vi "Cam prepare task.vi"(7 "save folder":path, 8 "error in (no error)":errorcluster, 10 "Cam task parameters":T1, 11 "Camera in":refnum<class "Camera.lvclass">) -> (0 "error out":errorcluster, 3 "Camera out":refnum<class "Camera.lvclass">)   [LabVIEW 2021, in "Camera.lvlib" / "Camera.lvclass"]
uses:
  Camera.lvclass
  C:/Program Files (x86)/National Instruments/LabVIEW 2021/vi.lib/ActorFramework/Actor/Actor.lvclass
  Cam task parameters.ctl
  Camera.lvclass/Camera.ctl
  <vilib>/ActorFramework/Actor/Actor.lvclass/Actor.ctl
  Main_Control/Main_Control Messages/UI change exposure time Msg/UI change exposure time Msg.lvclass/UI change exposure time Msg.ctl
  <vilib>/ActorFramework/Message Enqueuer/Message Enqueuer.lvclass/Message Enqueuer.ctl
  Main_Control/Main_Control/notifications.ctl
  Main_Control/Main_Control Messages/UI notifier Msg/UI notifier Msg.lvclass/UI notifier Msg.ctl
  <vilib>/ActorFramework/Message Enqueuer/Enqueue.vi
  Main_Control/Main_Control Messages/UI change exposure time Msg/UI change exposure time Msg.lvclass
  C:/Program Files (x86)/National Instruments/LabVIEW 2021/vi.lib/ActorFramework/Message/Message.lvclass
  Main_Control/Main_Control Messages/UI notifier Msg/UI notifier Msg.lvclass
  <vilib>/ActorFramework/Message Priority Queue/Priority Enqueue.vi
  <vilib>/ActorFramework/Actor/Actor.lvclass
  Main_Control/Main_Control/Main_Control.lvclass
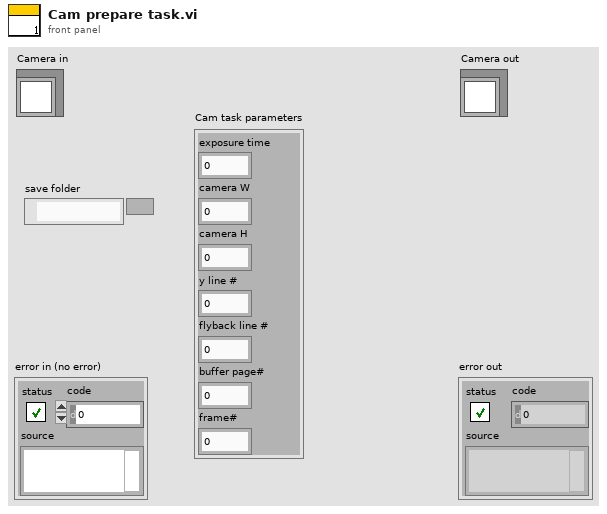
[diagram p1: front panel]
types:
  T1 = typedef "Camera.lvlib/Camera.lvclass/Cam task parameters.ctl" = cluster{"exposure time":dbl, "camera W":dbl, "camera H":dbl, "y line #":dbl, "flyback line #":dbl, "buffer page#":dbl, "frame#":dbl}
  T2 = cluster{"Horizontal Offset":i32, "Vertical Offset":i32, "Horizontal Size":i32, "Vertical Size":i32}
  T3 = typedef "Main_Control.lvlib/Main_Control.lvclass/notifications.ctl" = enum16{"cam 1 frame skkipped", "cam finish", "cam started", "cam stopped", "cam updated", "ni started", "ni stopped", "ni updated"}
  T4 = cluster{"Full Height":dbl, "Full Width":dbl, "Output Trigger Port":dbl}
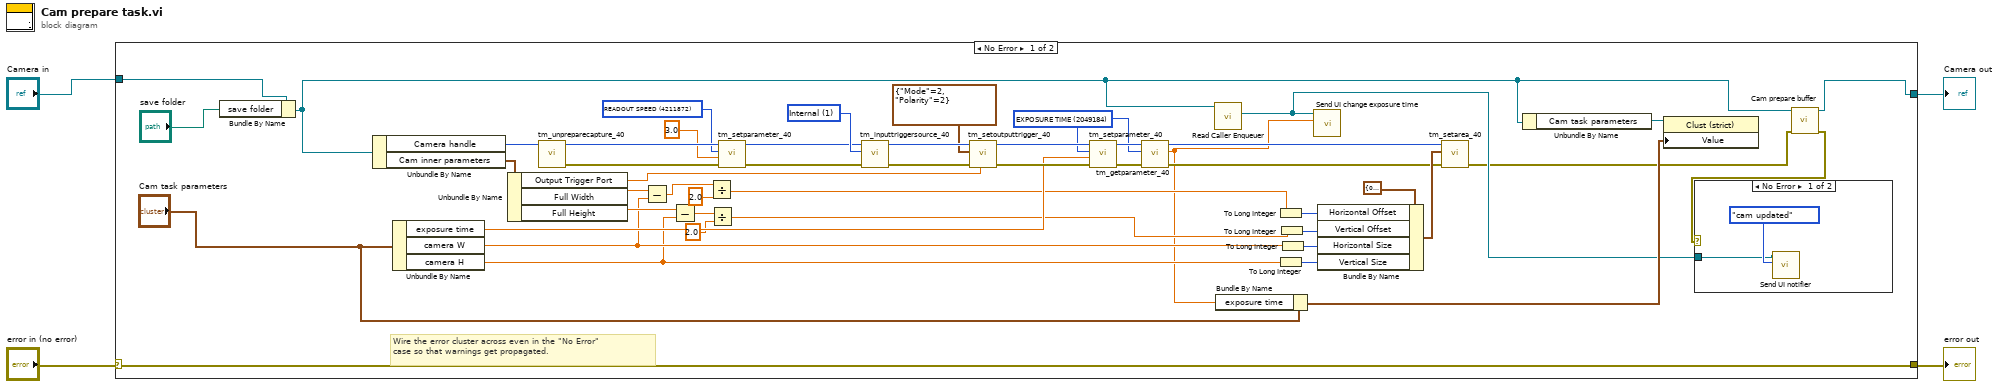
[diagram p0: block diagram]
diagram:
  n1 = case shown="No Error" "error in (no error)" {
    selector: "error in (no error)" -> [w9 w57]
    tunnel: [w9 w57] -> w3
    tunnel: [w7 w56] -> w1
    tunnel: "Camera in" -> [w14 w56]
    frame No Error {
      w34 = u32 2049184 items=["SENSOR MODE"=4212128, "READOUT SPEED"=4211872, "READOUT DIRECTION"=4211904, "TRIGGER GLOBAL EXPOSURE"=2049680, "TRIGGER DELAY"=1066480, "INTERNAL TRIGGER HANDLING"=1066496, "SYNC READOUT SYSTEM BLANK"=1066528, "SENSOR TEMPERATURE"=2115232, "SENSOR COOLER STATUS"=2115280, "EXPOSURE TIME"=2049184, "DEFECT CORRECT MODE"=4670368, "BINNING"=4215968, "INTERNAL LINE SPEED"=4226000, "INTERNAL LINE INTERVAL"=4226016, "NUMBER OF OUTPUT TRIGGER CONNECTOR"=1852320, "OUTPUT TRIGGER SOURCE[0]"=1852576, "OUTPUT TRIGGER SOURCE[1]"=1852832, "OUTPUT TRIGGER SOURCE[2]"=1853088, "OUTPUT TRIGGER POLARITY[0]"=1852592, "OUTPUT TRIGGER POLARITY[1]"=1852848, "OUTPUT TRIGGER POLARITY[2]"=1853104, "OUTPUT TRIGGER ACTIVE[0]"=1852608, "OUTPUT TRIGGER ACTIVE[1]"=1852864, "OUTPUT TRIGGER ACTIVE[2]"=1853120, "OUTPUT TRIGGER DELAY[0]"=1852624, "OUTPUT TRIGGER DELAY[1]"=1852880, "OUTPUT TRIGGER DELAY[2]"=1853136, "OUTPUT TRIGGER PERIOD[0]"=1852640, "OUTPUT TRIGGER PERIOD[1]"=1852896, "OUTPUT TRIGGER PERIOD[2]"=1853152, "OUTPUT TRIGGER KIND[0]"=1852656, "OUTPUT TRIGGER KIND[1]"=1852912, "OUTPUT TRIGGER KIND[2]"=1853168, "OUTPUT TRIGGER BASE SENSOR[0]"=1852672, "OUTPUT TRIGGER BASE SENSOR[1]"=1852928, "OUTPUT TRIGGER BASE SENSOR[2]"=1853184, "OUTPUT TRIGGER PRE HSYNC COUNT"=1852704] ("Parameter")
      w43 = u32 4211872 items=["SENSOR MODE"=4212128, "READOUT SPEED"=4211872, "READOUT DIRECTION"=4211904, "TRIGGER GLOBAL EXPOSURE"=2049680, "TRIGGER DELAY"=1066480, "INTERNAL TRIGGER HANDLING"=1066496, "SYNC READOUT SYSTEM BLANK"=1066528, "SENSOR TEMPERATURE"=2115232, "SENSOR COOLER STATUS"=2115280, "EXPOSURE TIME"=2049184, "DEFECT CORRECT MODE"=4670368, "BINNING"=4215968, "INTERNAL LINE SPEED"=4226000, "INTERNAL LINE INTERVAL"=4226016, "NUMBER OF OUTPUT TRIGGER CONNECTOR"=1852320, "OUTPUT TRIGGER SOURCE[0]"=1852576, "OUTPUT TRIGGER SOURCE[1]"=1852832, "OUTPUT TRIGGER SOURCE[2]"=1853088, "OUTPUT TRIGGER POLARITY[0]"=1852592, "OUTPUT TRIGGER POLARITY[1]"=1852848, "OUTPUT TRIGGER POLARITY[2]"=1853104, "OUTPUT TRIGGER ACTIVE[0]"=1852608, "OUTPUT TRIGGER ACTIVE[1]"=1852864, "OUTPUT TRIGGER ACTIVE[2]"=1853120, "OUTPUT TRIGGER DELAY[0]"=1852624, "OUTPUT TRIGGER DELAY[1]"=1852880, "OUTPUT TRIGGER DELAY[2]"=1853136, "OUTPUT TRIGGER PERIOD[0]"=1852640, "OUTPUT TRIGGER PERIOD[1]"=1852896, "OUTPUT TRIGGER PERIOD[2]"=1853152, "OUTPUT TRIGGER KIND[0]"=1852656, "OUTPUT TRIGGER KIND[1]"=1852912, "OUTPUT TRIGGER KIND[2]"=1853168, "OUTPUT TRIGGER BASE SENSOR[0]"=1852672, "OUTPUT TRIGGER BASE SENSOR[1]"=1852928, "OUTPUT TRIGGER BASE SENSOR[2]"=1853184, "OUTPUT TRIGGER PRE HSYNC COUNT"=1852704] ("Parameter")
      w50 = 1 items=["Internal"=1, "External"=2, "Software"=3, "Master Pulse"=4] ("Source")
      # "Wire the error cluster across even in the \"No Error\"\ncase so that warnings get propagated."
      n2 = Bundle By Name(cluster=w14, "save folder"="save folder") -> (w8:refnum<class "Camera.lvclass">)
      n3 = Unbundle By Name(w8) -> ("Camera handle"=w53:u32, "Cam inner parameters"=w32:T4)
      n4 = Unbundle By Name("Cam task parameters") -> ("exposure time"=w33:dbl, "camera W"=w23:dbl, "camera H"=w21:dbl)
      n5 = Unbundle By Name(w32) -> ("Output Trigger Port"=w17:dbl, "Full Width"=w30:dbl, "Full Height"=w31:dbl)
      n6 = call <userlib>:"tm_unpreparecapture_40.vi"("Handle in"=w53) -> ("error out"=w42:errorcluster, "Handle out"=w46:u32)  [unwired: 9 in]
      n7 = Subtract(x=w30, y=w23) -> (x-y=w26:dbl)
      n8 = Subtract(x=w31, y=w21) -> (x-y=w28:dbl)
      n9 = Divide(x=w26, y=2.0) -> (x/y=w19:dbl)
      n10 = Divide(x=w28, y=2.0) -> (x/y=w18:dbl)
      n11 = call <userlib>:"tm_setparameter_40.vi"("error in (no error)"=w42, "Value in"=3.0 ("Value"), "Parameter"=w43, "Handle in"=w46) -> ("error out"=w41:errorcluster, "Handle out"=w45:u32)  [unwired: 6 in]
      n12 = call <userlib>:"tm_inputtriggersource_40.vi"("error in (no error)"=w41, "Source"=w50, "Handle in"=w45) -> ("error out"=w51:errorcluster, "Handle out"=w52:u32)  [unwired: 7 in]
      n13 = call <userlib>:"tm_setoutputtrigger_40.vi"("Port"=w17, "error in (no error)"=w51, "Type"=cluster{"Mode":u32, "Polarity":u32} {"Mode"=2, "Polarity"=2}, "Handle in"=w52) -> ("error out"=w39:errorcluster, "Handle out"=w40:u32)  [unwired: 6 in]
      n14 = call <userlib>:"tm_setparameter_40.vi"("error in (no error)"=w39, "Value in"=w33, "Parameter"=w34, "Handle in"=w40) -> ("error out"=w36:errorcluster, "Handle out"=w38:u32)  [unwired: 6 in]
      n15 = call <userlib>:"tm_getparameter_40.vi"("error in (no error)"=w36, "Parameter"=w34, "Handle in"=w38) -> ("error out"=w35:errorcluster, "Value out"=w12:dbl, "Handle out"=w37:u32)  [unwired: 6 in]
      n16 = call <vilib>:"Read Caller Enqueuer.vi"("Actor"=w8) -> ("Caller Enqueuer"=w11:refnum<class "Message Enqueuer.lvclass">)  [unwired: 10 in]
      n17 = Bundle By Name(cluster="Cam task parameters", "exposure time"=w12) -> (w15:T1)
      n18 = To Long Integer(number=w19) -> (32bit integer=w25:i32)
      n19 = To Long Integer(number=w21) -> (32bit integer=w20:i32)
      n20 = To Long Integer(number=w18) -> (32bit integer=w24:i32)
      n21 = To Long Integer(number=w23) -> (32bit integer=w22:i32)
      n22 = call "Send UI change exposure time.vi"("exposure time"=w12, "Message Enqueuer"=w11) -> ()  [unwired: 8 in, 2 out]
      n23 = Bundle By Name(cluster=T2 {"Horizontal Offset"=0, "Vertical Offset"=0, "Horizontal Size"=0, "Vertical Size"=0} ("Sub Region"), "Horizontal Offset"=w25, "Vertical Offset"=w24, "Horizontal Size"=w22, "Vertical Size"=w20) -> (w48:T2)
      n24 = call <userlib>:"tm_setarea_40.vi"("error in (no error)"=w35, "Sub Region"=w48, "Handle in"=w37) -> ("error out"=w6:errorcluster)  [unwired: 7 in, 1 out]
      n25 = Unbundle By Name(w8) -> ("Cam task parameters"=w10:refnum<vi>)
      n26 = property class="Clust (strict)"(reference=w10, "Value"=w15) -> ()  [unwired: 1 in, 2 out]
      n27 = call "Cam prepare buffer.vi"("error in (no error)"=w6, "Camera in"=w8) -> ("error out"=w5:errorcluster, "Camera out"=w7:refnum<class "Camera.lvclass">)  [unwired: 8 in]
      n28 = case shown="No Error" w5 {
        tunnel: w11 -> [w54 _]
        frame No Error {
          n29 = call "Send UI notifier.vi"("Object&State"=notifications."cam updated", "Message Enqueuer"=w54) -> ()  [unwired: 8 in, 2 out]
        }
        frame Error {
        }
      }
    }
    frame Error {
    }
  }
  "error out" <- w3
  "Camera out" <- w1
